vi "u(t)76R.vi"(5 "Desire Velosity":dbl(slide) scale=-10.0..10.0, 6 "Velocity":dbl) -> (1 "u(t)":dbl)   [LabVIEW 2018]
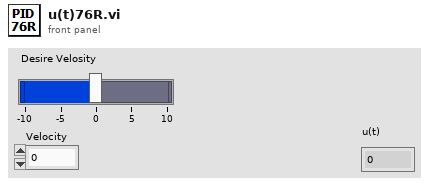
[diagram p1: front panel]
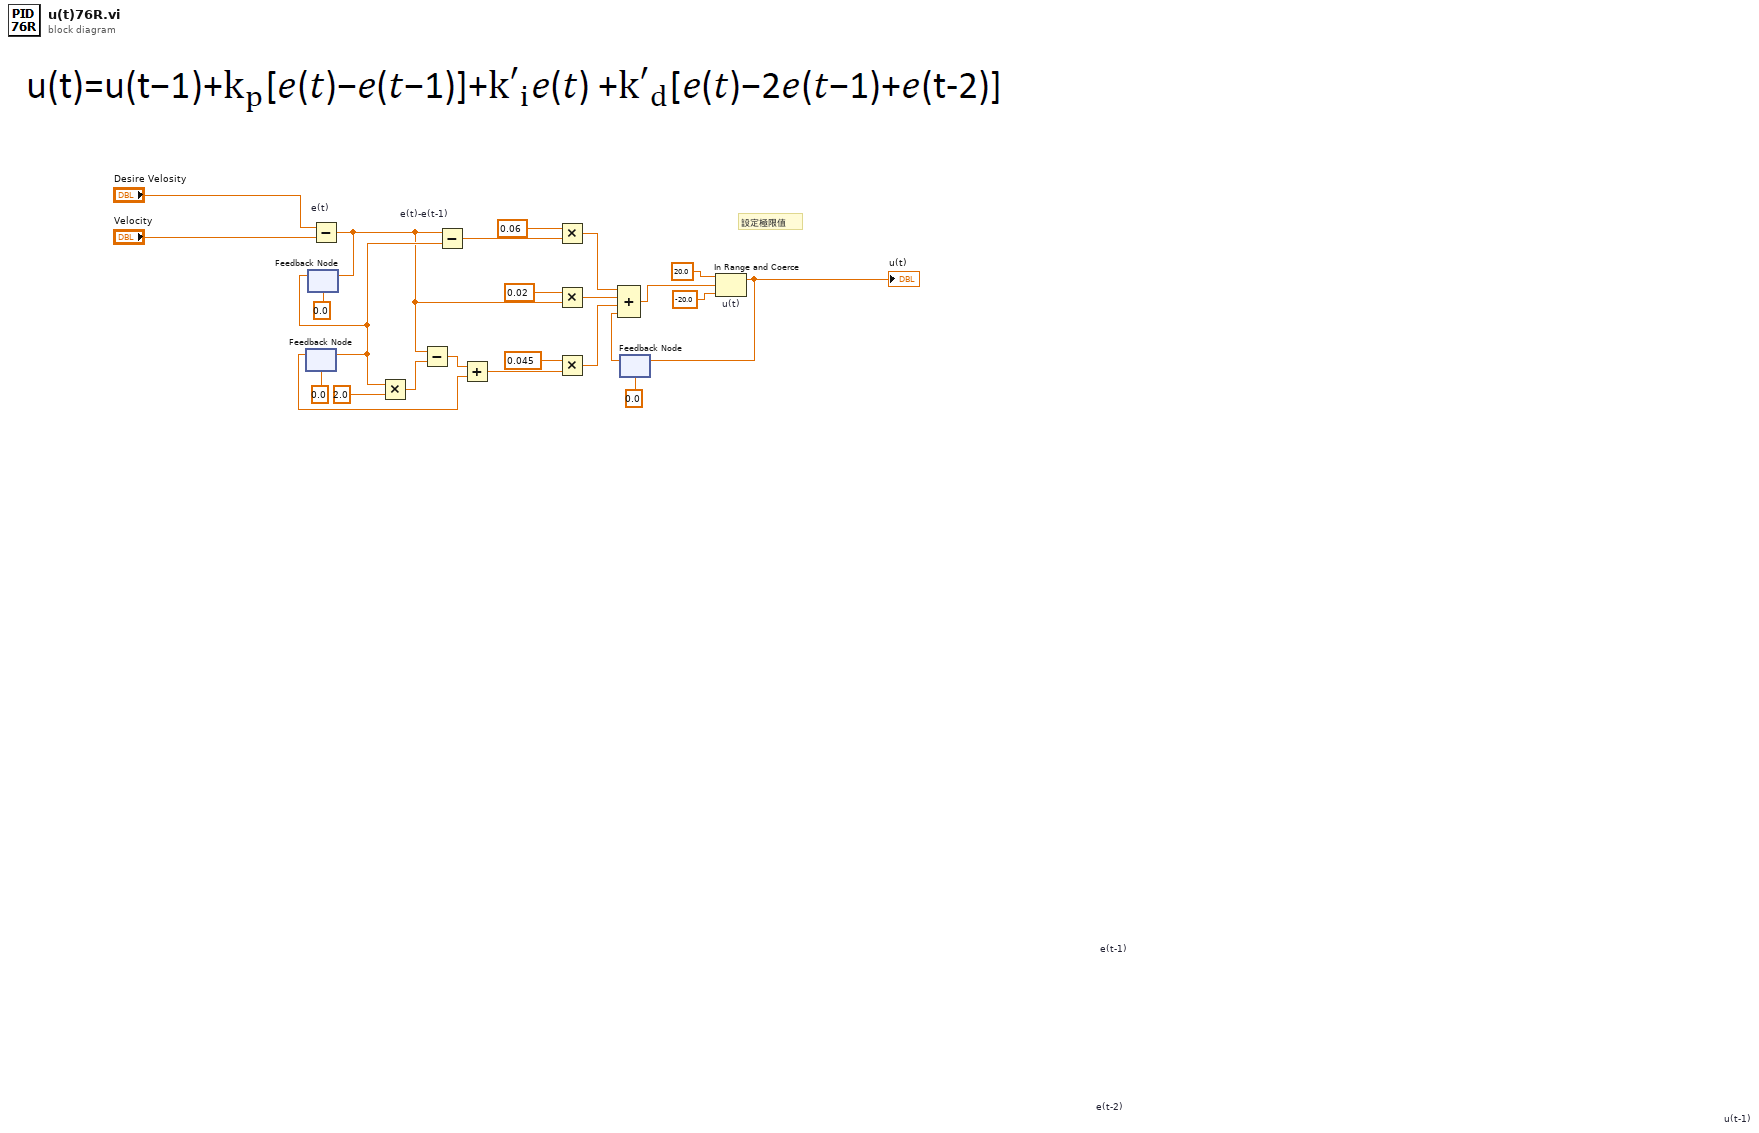
[diagram p0: block diagram]
diagram:
  # "設定極限值"
  n1 = feedback #1 "e(t-2)"(0.0) -> (w13:dbl)
  n2 = feedback #2 "e(t-1)"(0.0) -> (w4:dbl)
  n3 = feedback-in #1(w4) -> ()
  n4 = Subtract "e(t)"(x="Desire Velosity", y="Velocity") -> (x-y=w3:dbl)
  n5 = feedback-in #2(w3) -> ()
  n6 = Multiply(x=w4, y=2.0) -> (x*y=w11:dbl)
  n7 = Subtract(x=w3, y=w11) -> (x-y=w12:dbl)
  n8 = Subtract "e(t)-e(t-1)"(x=w3, y=w4) -> (x-y=w7:dbl)
  n9 = Add(x=w12, y=w13) -> (x+y=w14:dbl)
  n10 = Multiply(x=0.06 ("Kp"), y=w7) -> (x*y=w16:dbl)
  n11 = Multiply(x=0.02 ("Ki"), y=w3) -> (x*y=w17:dbl)
  n12 = Multiply(x=0.045 ("Kd"), y=w14) -> (x*y=w18:dbl)
  n13 = feedback #3 "u(t-1)"(0.0) -> (w19:dbl)
  n14 = Compound Arithmetic op=ADD(w16, w17, w18, w19) -> (w21:dbl)
  n15 = In Range and Coerce "u(t)"(upper limit=20.0, x=w21, lower limit=-20.0 ("y")) -> (coerced(x)=w24:dbl)  [unwired: 1 out]
  "u(t)" <- w24
  n16 = feedback-in #3(w24) -> ()
